vi "Default Settings.vi"() -> (3 "Default Settings":T1={"TDMS Filepath"=path "", "TDMS Directory"=path "", "Dir?"=TRUE})   [LabVIEW 2019, in "Filepath Editor.lvlib"]
doc: "_____\nBased on DQMH Project Template 6.1.0.94."
uses:
  Filepath Editor.lvlib
  Settings--cluster.ctl
  <vilib>/Utility/sysdir.llb/System Directory Type.ctl
panel:
  out "appended path":path
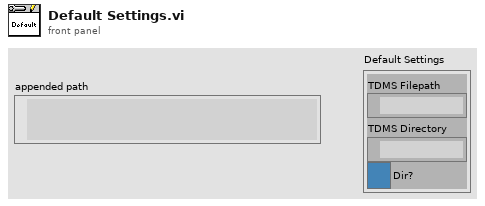
[diagram p1: front panel]
types:
  T1 = typedef "Filepath Editor.lvlib/Settings--cluster.ctl" = cluster{"TDMS Filepath":path, "TDMS Directory":path, "Dir?":bool}
  T2 = typedef "System Directory Type.ctl" = i32
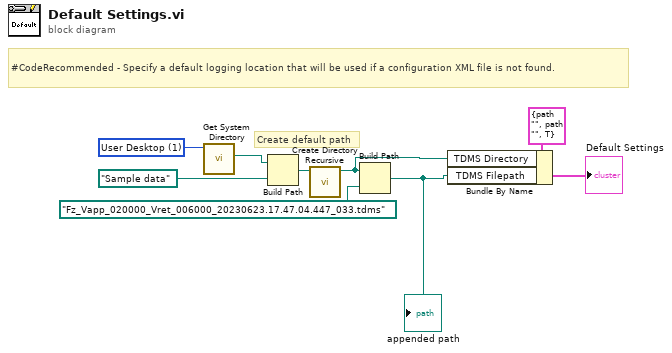
[diagram p0: block diagram]
diagram:
  w9 = T2 1 items=["User Home"=0, "User Desktop"=1, "User Documents"=2, "User Application Data"=3, "User Preferences"=4, "User Temporary"=5, "Public Documents"=6, "Public Application Data"=7, "Public Preferences"=8, "Public Cache"=13, "System Core Libraries"=9, "System Installed Libraries"=10, "Application Files"=11, "Boot Volume Root"=12] ("system directory type")
  # "#CodeRecommended - Specify a default logging location that will be used if a configuration XML file is not found."
  # "Create default path"
  n1 = call <vilib>:"Get System Directory.vi"("system directory type"=w9) -> ("system directory"=w8:path)  [unwired: 10 in]
  n2 = Build Path(base path=w8, name or relative path=path "Sample data") -> (appended path=w7:path)
  n3 = call <vilib>:"Create Directory Recursive.vi"("directory"=w7) -> ("directory copy"=w1:path)  [unwired: 4 in, 2 out]
  n4 = Build Path(base path=w1, name or relative path=path "Fz_Vapp_020000_Vret_006000_20230623.17.47.04.447_033.tdms") -> (appended path=w2:path)
  "appended path" <- w2
  n5 = Bundle By Name(cluster=T1 {"TDMS Filepath"=path "", "TDMS Directory"=path "", "Dir?"=TRUE} ("Default Settings"), "TDMS Directory"=w1, "TDMS Filepath"=w2) -> (→"Default Settings":T1)
